vi "In_S2F33.vi"(8 "error in (no error)":errorcluster, 11 "S2 Message Class in":refnum<class "S2 Message Class.lvclass">) -> (0 "error out":errorcluster, 1 "OK?":bool, 2 "S2F33":T1, 3 "S2 Message Class out":refnum<class "S2 Message Class.lvclass">)   [LabVIEW 2020, in "SECS Communication.lvlib" / "S2 Message Class.lvclass"]
uses:
  S2 Message Class.lvclass
  D:/Dropbox/SECS/SECS_GEM v1.0.6/Com/SECS Communication/SECS-II Class/SECS-II Class.lvclass
  S2F33.ctl
  SECS-II Class/SECS-II Class.lvclass/SECS-II Class.ctl
  SECS-II Class/Variant To Data_U4.vi
  SECS-II Class/Variant To Data_ASCII.vi
  SECS-II Class/Variant To Data_I1.vi
  SECS-II Class/Variant To Data_I2.vi
  SECS-II Class/Variant To Data_I4.vi
  SECS-II Class/Variant To Data_I8.vi
  SECS-II Class/Variant To Data_U1.vi
  SECS-II Class/Variant To Data_U2.vi
  SECS-II Class/Variant To Data_U8.vi
  SECS-II Class/SECS-II Class.lvclass
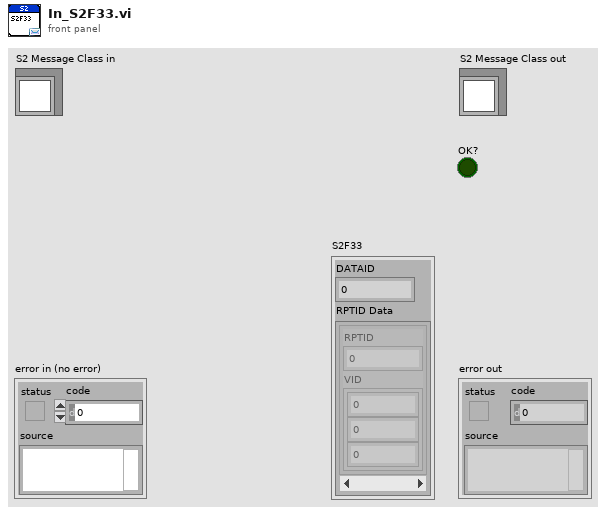
[diagram p1: front panel]
types:
  T1 = typedef "SECS Communication.lvlib/S2 Message Class.lvclass/S2F33.ctl" = cluster{"DATAID":u32, "RPTID Data":cluster{"RPTID":u32, "VID":u32[]}[]}
  T2 = typedef "SECS Communication.lvlib/SECS-II Class.lvclass/Message Data.ctl" = cluster{"Index":i32, "Data Item Format":T3, "Format Code":T4, "Parent Index":i32, "Child Index":i32[], "Data":variant}
  T3 = typedef "SECS Communication.lvlib/SECS-II Class.lvclass/Data Item Format.ctl" = enum16{"Data Type", "Value"}
  T4 = typedef "SECS Communication.lvlib/SECS-II Class.lvclass/Format Code.ctl" = enum16{"L", "A", "B", "Boolean", "J", "I1", "I2", "I4", "I8", "U1", "U2", "U4", "U8", "F4", "F8", "Char"}
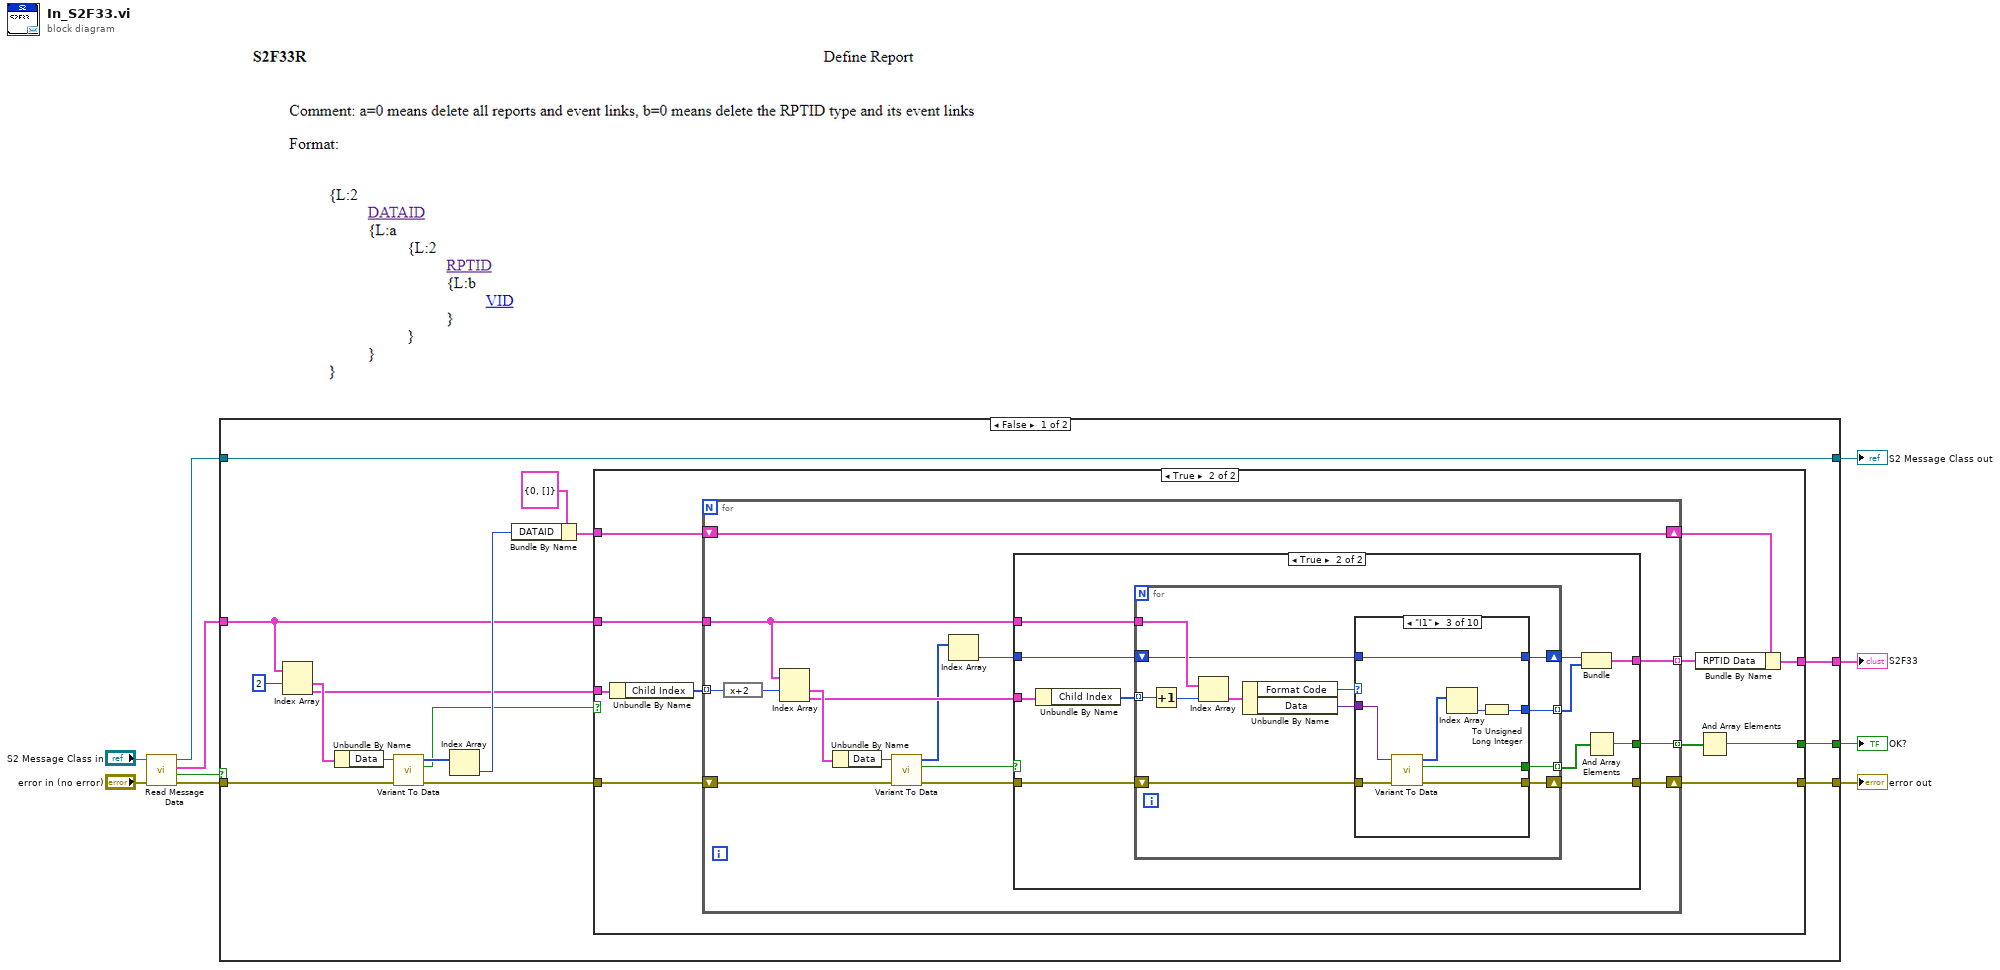
[diagram p0: block diagram]
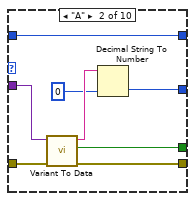
[diagram p5: hidden frame]
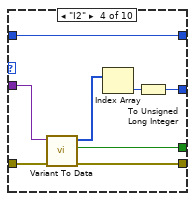
[diagram p6: hidden frame]
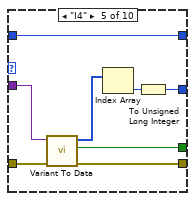
[diagram p7: hidden frame]
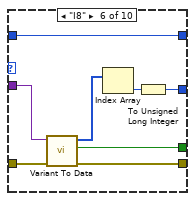
[diagram p8: hidden frame]
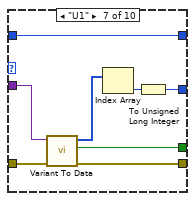
[diagram p9: hidden frame]
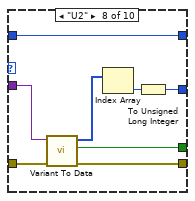
[diagram p10: hidden frame]
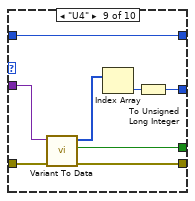
[diagram p11: hidden frame]
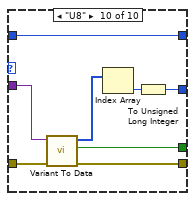
[diagram p12: hidden frame]
diagram:
  n1 = call "Read Message Data.vi"("error in (no error)"="error in (no error)", "SECS-II Class in"="S2 Message Class in") -> ("error out"=w10:errorcluster, "Empty?"=w9:bool, "Message Data"=w7:T2[], "SECS-II Class out"=w8:refnum<class "S2 Message Class.lvclass">)  [unwired: 6 in]
  n2 = case shown="False" w9 {
    tunnel: w10 -> [w24 w152]
    tunnel: w8 -> [w14 w153]
    tunnel: w7 -> [w15 _]
    tunnel: [w14 w153] -> w5
    tunnel: [w13 w152] -> w6
    tunnel: [w12 _] -> w4
    tunnel: [w11 _] -> w3
    frame False {
      n3 = Index Array(array=w15, index #1=2 ("index")) -> (element #1=w25:T2, element #2=w16:T2)  [unwired: 1 in]
      n4 = Unbundle By Name(w25) -> ("Data"=w23:variant)
      n5 = call-poly "Variant To Data.vi"("error in (no error)"=w24, "Variant"=w23) -> ("error out"=w19:errorcluster, "OK?"=w18:bool, "Data"=w21:u32[])  [unwired: 7 in]
      n6 = Index Array(array=w21) -> (element=w20:u32)  [unwired: 1 in]
      n7 = Bundle By Name(cluster=T1 {"DATAID"=0, "RPTID Data"=[]} ("S2F33"), "DATAID"=w20) -> (w17:T1)
      n8 = case shown="True" w18 {
        tunnel: w19 -> [w27 w36]
        tunnel: w17 -> [_ w32]
        tunnel: w16 -> [_ w38]
        tunnel: w15 -> [_ w35]
        tunnel: [w27 w30] -> w13
        tunnel: [_ w29] -> w12
        tunnel: [_ w28] -> w11
        frame False {
        }
        frame True {
          n9 = Unbundle By Name(w38) -> ("Child Index"=w37:i32[])
          n10 = for {
            tunnel: w37 -> [w40] mode=indexing
            shift-right: [w43] -> w30
            shift-left: w36 -> [w52]
            tunnel: w35 -> [w47]
            tunnel: [w44] -> w34 mode=indexing
            tunnel: [w42] -> w33 mode=indexing
            shift-right: [w41] -> w31
            shift-left: w32 -> [w41]
            n11 = expression code="x+2"(w40) -> (w39:i32)
            n12 = Index Array(array=w47, index #1=w39) -> (element #1=w51:T2, element #2=w48:T2)  [unwired: 1 in]
            n13 = Unbundle By Name(w51) -> ("Data"=w53:variant)
            n14 = call-poly "Variant To Data.vi"("error in (no error)"=w52, "Variant"=w53) -> ("error out"=w50:errorcluster, "OK?"=w49:bool, "Data"=w46:u32[])  [unwired: 7 in]
            n15 = Index Array(array=w46) -> (element=w45:u32)  [unwired: 1 in]
            n16 = case shown="True" w49 {
              tunnel: w50 -> [w54 w64]
              tunnel: w48 -> [_ w65]
              tunnel: w47 -> [_ w62]
              tunnel: w45 -> [_ w61]
              tunnel: [_ w57] -> w44
              tunnel: [_ w56] -> w42
              tunnel: [w54 w55] -> w43
              frame False {
              }
              frame True {
                n17 = Unbundle By Name(w65) -> ("Child Index"=w63:i32[])
                n18 = for {
                  shift-right: [w68] -> w55
                  shift-left: w64 -> [w69]
                  tunnel: w63 -> [w77] mode=indexing
                  tunnel: w62 -> [w76]
                  shift-right: [w70] -> w60
                  shift-left: w61 -> [w71]
                  tunnel: [w67] -> w58 mode=indexing
                  tunnel: [w66] -> w59 mode=indexing
                  n19 = Increment(x=w77) -> (x+1=w75:i32)
                  n20 = Index Array(array=w76, index=w75) -> (element=w74:T2)
                  n21 = Unbundle By Name(w74) -> ("Format Code"=w73:T4, "Data"=w72:variant)
                  n22 = case shown="\"I1\"" w73 {
                    tunnel: w72 -> [_ w85 w93 w101 w109 w117 w125 w133 w141 w149]
                    tunnel: w71 -> [w79 w87 w95 w103 w111 w119 w127 w135 w143 w151]
                    tunnel: [w79 w87 w95 w103 w111 w119 w127 w135 w143 w151] -> w70
                    tunnel: w69 -> [w78 w86 w94 w102 w110 w118 w126 w134 w142 w150]
                    tunnel: [w78 w84 w92 w100 w108 w116 w124 w132 w140 w148] -> w68
                    tunnel: [_ w83 w91 w96 w104 w112 w120 w128 w136 w144] -> w67
                    tunnel: [_ w80 w89 w98 w106 w114 w122 w130 w138 w146] -> w66
                    frame Default {
                    }
                    frame "A" {
                      n23 = call-poly "Variant To Data.vi"("error in (no error)"=w86, "Variant"=w85) -> ("error out"=w84:errorcluster, "OK?"=w83:bool, "Data"=w82:string)  [unwired: 7 in]
                      n24 = Decimal String To Number(string=w82, default (0L)=u32 0 ("default (0 I32)")) -> (number=w80:u32)  [unwired: 1 in, 1 out]
                    }
                    frame "I1" {
                      n25 = call-poly "Variant To Data.vi"("error in (no error)"=w94, "Variant"=w93) -> ("error out"=w92:errorcluster, "OK?"=w91:bool, "Data"=w88:i8[])  [unwired: 7 in]
                      n26 = Index Array(array=w88) -> (element=w90:i8)  [unwired: 1 in]
                      n27 = To Unsigned Long Integer(number=w90) -> (unsigned 32bit integer=w89:u32)
                    }
                    frame "I2" {
                      n28 = call-poly "Variant To Data.vi"("error in (no error)"=w102, "Variant"=w101) -> ("error out"=w100:errorcluster, "OK?"=w96:bool, "Data"=w97:i16[])  [unwired: 7 in]
                      n29 = Index Array(array=w97) -> (element=w99:i16)  [unwired: 1 in]
                      n30 = To Unsigned Long Integer(number=w99) -> (unsigned 32bit integer=w98:u32)
                    }
                    frame "I4" {
                      n31 = call-poly "Variant To Data.vi"("error in (no error)"=w110, "Variant"=w109) -> ("error out"=w108:errorcluster, "OK?"=w104:bool, "Data"=w105:i32[])  [unwired: 7 in]
                      n32 = Index Array(array=w105) -> (element=w107:i32)  [unwired: 1 in]
                      n33 = To Unsigned Long Integer(number=w107) -> (unsigned 32bit integer=w106:u32)
                    }
                    frame "I8" {
                      n34 = call-poly "Variant To Data.vi"("error in (no error)"=w118, "Variant"=w117) -> ("error out"=w116:errorcluster, "OK?"=w112:bool, "Data"=w113:i64[])  [unwired: 7 in]
                      n35 = Index Array(array=w113) -> (element=w115:i64)  [unwired: 1 in]
                      n36 = To Unsigned Long Integer(number=w115) -> (unsigned 32bit integer=w114:u32)
                    }
                    frame "U1" {
                      n37 = call-poly "Variant To Data.vi"("error in (no error)"=w126, "Variant"=w125) -> ("error out"=w124:errorcluster, "OK?"=w120:bool, "Data"=w121:u8[])  [unwired: 7 in]
                      n38 = Index Array(array=w121) -> (element=w123:u8)  [unwired: 1 in]
                      n39 = To Unsigned Long Integer(number=w123) -> (unsigned 32bit integer=w122:u32)
                    }
                    frame "U2" {
                      n40 = call-poly "Variant To Data.vi"("error in (no error)"=w134, "Variant"=w133) -> ("error out"=w132:errorcluster, "OK?"=w128:bool, "Data"=w129:u16[])  [unwired: 7 in]
                      n41 = Index Array(array=w129) -> (element=w131:u16)  [unwired: 1 in]
                      n42 = To Unsigned Long Integer(number=w131) -> (unsigned 32bit integer=w130:u32)
                    }
                    frame "U4" {
                      n43 = call-poly "Variant To Data.vi"("error in (no error)"=w142, "Variant"=w141) -> ("error out"=w140:errorcluster, "OK?"=w136:bool, "Data"=w137:u32[])  [unwired: 7 in]
                      n44 = Index Array(array=w137) -> (element=w139:u32)  [unwired: 1 in]
                      n45 = To Unsigned Long Integer(number=w139) -> (unsigned 32bit integer=w138:u32)
                    }
                    frame "U8" {
                      n46 = call-poly "Variant To Data.vi"("error in (no error)"=w150, "Variant"=w149) -> ("error out"=w148:errorcluster, "OK?"=w144:bool, "Data"=w145:u64[])  [unwired: 7 in]
                      n47 = Index Array(array=w145) -> (element=w147:u64)  [unwired: 1 in]
                      n48 = To Unsigned Long Integer(number=w147) -> (unsigned 32bit integer=w146:u32)
                    }
                  }
                }
                n49 = Bundle("Data"=w60, w59) -> (w56:cluster{"Data":u32, u32[]})  [unwired: 1 in]
                n50 = And Array Elements(Boolean array=w58) -> (logical AND=w57:bool)
              }
            }
          }
          n51 = Bundle By Name(cluster=w31, "RPTID Data"=w33) -> (w29:T1)
          n52 = And Array Elements(Boolean array=w34) -> (logical AND=w28:bool)
        }
      }
    }
    frame True {
    }
  }
  "error out" <- w6
  "S2 Message Class out" <- w5
  "S2F33" <- w4
  "OK?" <- w3
